vi "Close.vi"(8 "error in (no error)":errorcluster, 11 "VISA resource name":refnum<visa-resource-name>) -> (0 "error out":errorcluster)   [LabVIEW 2020, in "ChromTech Series I Drivers.lvlib"]
doc: "Terminates the software connection to the instrument. This node runs normally even if an error occurred before this node runs."
uses:
  <instrlib>/RxnRover/ChromtechSeriesIDriver/ChromTech Series I Drivers.lvlib
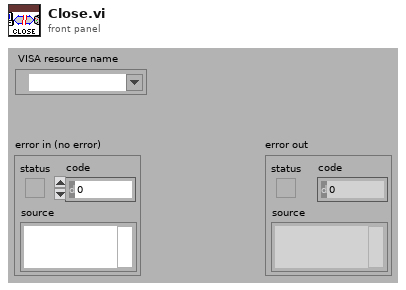
[diagram p1: front panel]
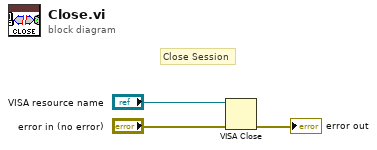
[diagram p0: block diagram]
diagram:
  # "Close Session"
  n1 = VISA Close(VISA resource name="VISA resource name", error in (no error)="error in (no error)") -> (error out=→"error out":errorcluster)
